vi "Get Number of Channels.vi"(8 "error in (no error)":errorcluster, 11 "DAQmx in":refnum<class "DAQmx.lvclass">) -> (0 "error out":errorcluster, 1 "Total Channels":u32, 2 "Channels each Device":u32[](array[numeric]), 3 "DAQmx out":refnum<class "DAQmx.lvclass">)   [LabVIEW 2019, in "DAQmx.lvclass"]
uses:
  DAQmx.lvclass
  DAQmx.lvclass/DAQmx.ctl
  <resource>/objmgr/daqmx.rc
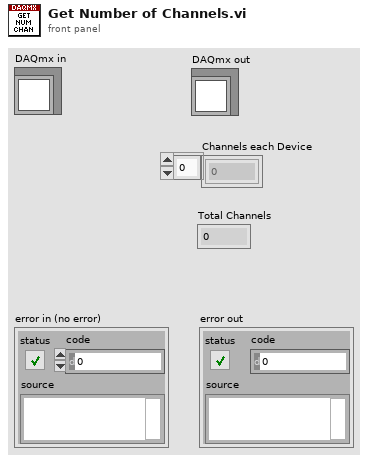
[diagram p1: front panel]
types:
  T1 = typedef "DAQmx.lvclass/DAQ.Config.AO--Cluster--Array.ctl" = T2[]
  T2 = typedef "DAQmx.lvclass/DAQ.Config.AO--Cluster.ctl" = cluster{"Channels":tag, "Range":T3, "output terminal configuration":i32, "Type":T4}
  T3 = typedef "DAQmx.lvclass/DAQ.Config.AO.Range--enum.ctl" = enum16{"±0.1", "±1.0", "±3.5", "±10.0", ""}
  T4 = typedef "DAQmx.lvclass/DAQ.Config.Device Type--enum.ctl" = enum16{"None", "USB-4431", "PXI-446x"}
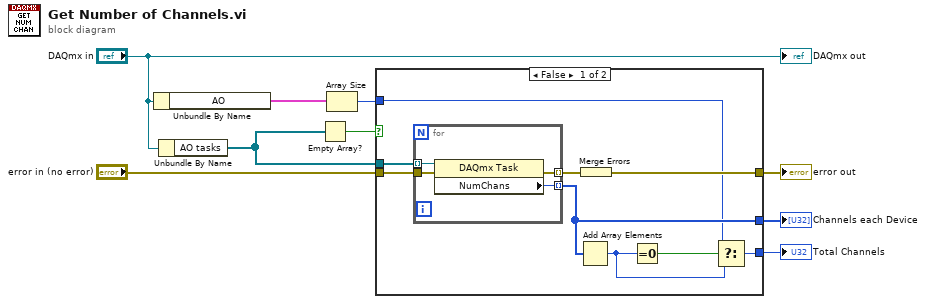
[diagram p0: block diagram]
diagram:
  n1 = Unbundle By Name("DAQmx in") -> ("AO"=w3:T1)
  n2 = Unbundle By Name("DAQmx in") -> ("AO tasks"=w2:refnum<k21>[])
  n3 = Empty Array?(array=w2) -> (empty?=w1:bool)
  n4 = Array Size(array=w3) -> (size(s)=w4:i32)
  n5 = case shown="False" w1 {
    tunnel: [w18 w24] -> w9
    tunnel: "error in (no error)" -> [w16 w24]
    tunnel: [w15 _] -> w7
    tunnel: [w13 w23] -> w5
    tunnel: w4 -> [w10 w23]
    tunnel: w2 -> [w11 _]
    frame False {
      n6 = for {
        tunnel: w11 -> [w22] mode=indexing
        tunnel: [w21] -> w15 mode=indexing
        tunnel: [w20] -> w17 mode=indexing
        tunnel: w16 -> [w19]
        n7 = property class="DAQmx Task"(reference=w22, error in=w19) -> (error out=w20:errorcluster, "NumChans"=w21:u32)  [unwired: 1 out]
      }
      n8 = Add Array Elements(numeric array=w15) -> (sum=w12:u32)
      n9 = Merge Errors(w17) -> (w18:errorcluster)
      n10 = Equal To 0?(x=w12) -> (x = 0?=w14:bool)
      n11 = Select(t=w10, s=w14, f=w12) -> (s? t:f=w13:u32)
    }
    frame True {
    }
  }
  "Total Channels" <- w5
  "error out" <- w9
  "Channels each Device" <- w7
  "DAQmx out" <- "DAQmx in"
